vi "LS330_LoopError.vi"(8 "error in":errorcluster) -> (2 "T button?":bool)   [LabVIEW 2021]
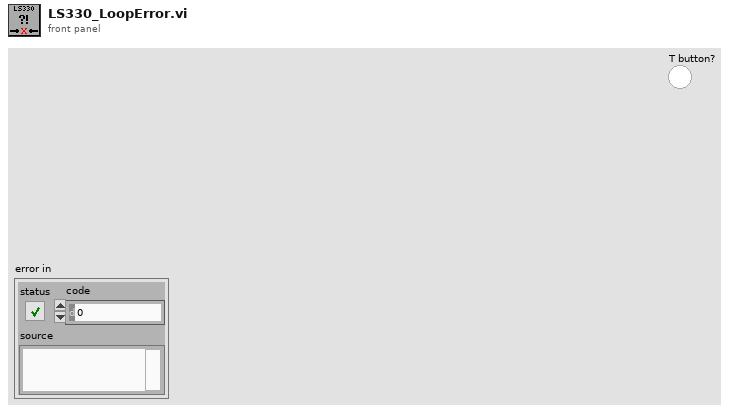
[diagram p1: front panel]
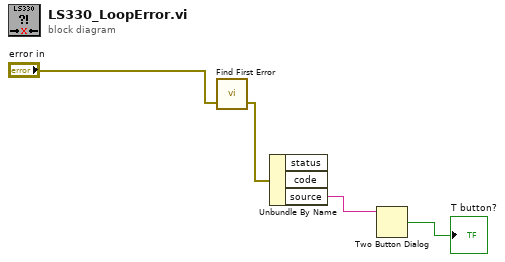
[diagram p0: block diagram]
diagram:
  n1 = call <vilib>:"Find First Error.vi"("error in (no error)"="error in") -> ("error out"=w3:errorcluster)  [unwired: 3 in, 1 out]
  n2 = Unbundle By Name(w3) -> ("source"=w2:string)  [unwired: 2 out]
  n3 = Two Button Dialog(message=w2) -> (T button?=→"T button?":bool)  [unwired: 2 in]
